vi "Read Cluster Size.vi"(8 "error in (no error)":errorcluster, 11 "Cluster.lvclass in":refnum<class "Cluster.lvclass">) -> (0 "error out":errorcluster, 2 "ClusterSize":T1, 3 "Cluster.lvclass out":refnum<class "Cluster.lvclass">)   [LabVIEW 2015, in "Cluster.lvclass"]
uses:
  Cluster.lvclass
  <vilib>/Utility/miscctls.llb/LVBoundsTypeDef.ctl
  Cluster.lvclass/Cluster.ctl
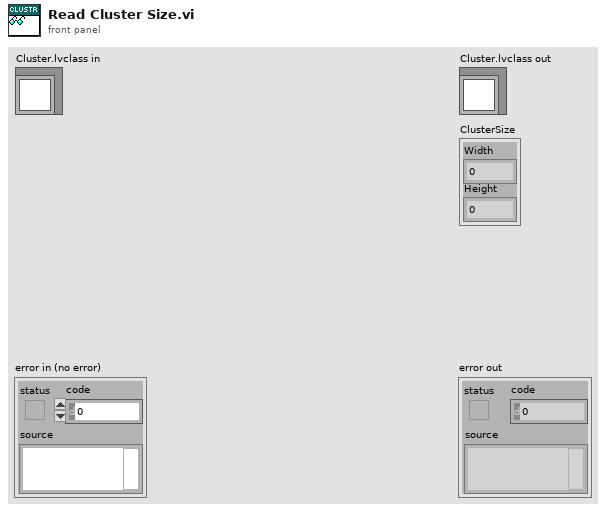
[diagram p1: front panel]
types:
  T1 = typedef "LVBoundsTypeDef.ctl" = cluster{"Width":u32, "Height":u32}
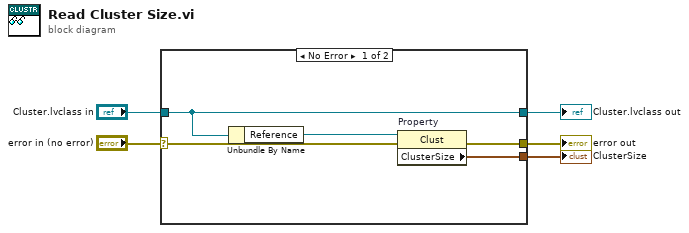
[diagram p0: block diagram]
diagram:
  n1 = case shown="No Error" "error in (no error)" {
    selector: "error in (no error)" -> [w6 w12]
    tunnel: [w9 w12] -> w4
    tunnel: [w8 w11] -> w2
    tunnel: "Cluster.lvclass in" -> [w8 w11]
    tunnel: [w10 _] -> w1
    frame No Error {
      n2 = Unbundle By Name(w8) -> ("Reference"=w7:refnum<vi>)
      n3 = property on="Property" class="Clust"(reference=w7, error in=w6) -> (error out=w9:errorcluster, "ClusterSize"=w10:T1)  [unwired: 1 out]
    }
    frame Error {
    }
  }
  "error out" <- w4
  "Cluster.lvclass out" <- w2
  "ClusterSize" <- w1
